vi "Configure Power Alternate.vi"(6 "Enable Alternate Amplitude (F: Disable)":bool, 7 "Trigger Source (0: Internal)":i32(ring) items=["Internal", "External"], 8 "error in (no error)":errorcluster, 9 "External Trigger Source (0: BBTrigger1)":i32(ring) items=["BBTrigger1", "BBTrigger2", "PTrig", "Event1"], 10 "Alternate Amplitude Delta Value (0 dB)":dbl, 11 "VISA resource name":refnum<visa-resource-name>) -> (0 "error out":errorcluster, 3 "VISA resource name out":refnum<visa-resource-name>)   [LabVIEW 2012, in "Agilent PSG MXG Series.lvlib"]
doc: "Configure alternate amplitude settings.\n\n<B>Notes:</B>\n(1) This VI is valid only in N5172B, N5182B."
uses:
  <instrlib>/Agilent PSG MXG Series/Agilent PSG MXG Series.lvlib
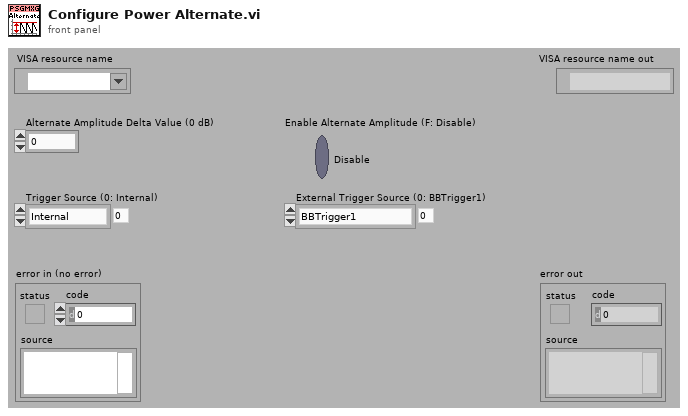
[diagram p1: front panel]
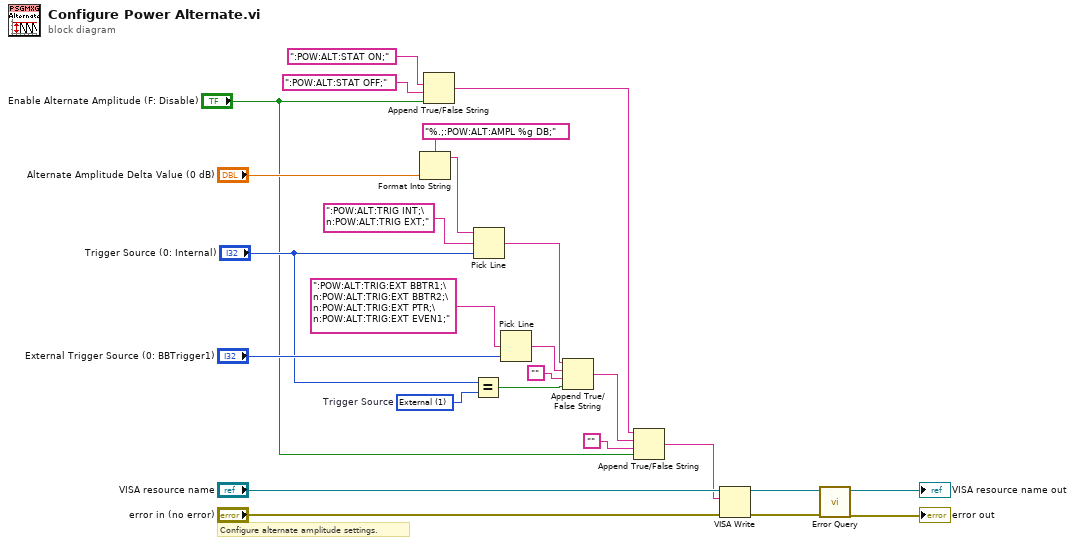
[diagram p0: block diagram]
diagram:
  w10 = 1 items=["Internal", "External"]  # Trigger Source
  # "Configure alternate amplitude settings."
  n1 = Format Into String(format string="%.;:POW:ALT:AMPL %g DB;", "Alternate Amplitude Delta Value (0 dB)") -> (resulting string=w12:string)  [unwired: 2 in, 1 out]
  n2 = Append True/False String(1:"Enable Alternate Amplitude (F: Disable)", 2:":POW:ALT:STAT OFF;", 3:":POW:ALT:STAT ON;") -> (0:w3:string)  [unwired: 1 out]
  n3 = Equal?(x="Trigger Source (0: Internal)", y=w10) -> (x = y?=w11:bool)
  n4 = Pick Line(string ("")=w12, multi-line string=":POW:ALT:TRIG INT;\n:POW:ALT:TRIG EXT;", line index="Trigger Source (0: Internal)") -> (output string=w6:string)
  n5 = Pick Line(multi-line string=":POW:ALT:TRIG:EXT BBTR1;\n:POW:ALT:TRIG:EXT BBTR2;\n:POW:ALT:TRIG:EXT PTR;\n:POW:ALT:TRIG:EXT EVEN1;", line index="External Trigger Source (0: BBTrigger1)") -> (output string=w8:string)  [unwired: 1 out]
  n6 = Append True/False String(1:w11, 2:"", 3:w8, 4:w6) -> (0:w4:string)
  n7 = Append True/False String(1:"Enable Alternate Amplitude (F: Disable)", 2:"", 3:w4, 4:w3) -> (0:w1:string)
  n8 = VISA Write(VISA resource name="VISA resource name", write buffer=w1, error in (no error)="error in (no error)") -> (VISA resource name out=w16:refnum<visa-resource-name>, error out=w15:errorcluster)  [unwired: 1 out]
  n9 = call <instrlib>:"Error Query.vi"("error in (no error)"=w15, "VISA resource name"=w16) -> ("error out"=→"error out":errorcluster, "VISA resource name out"=→"VISA resource name out":refnum<visa-resource-name>)  [unwired: 8 out]
